vi "Simulation Statechart -DLL Wrapper.vi"(5 "firstStep?":bool, 7 "enableVisualization?":bool=TRUE, 8 "error in":errorcluster, 10 "sensors":T1 {"Kobuki Sensors"."Charger Source" items=["DISCHARGING"=0, "DOCKING_CHARGED"=2, "DOCKING_CHARGING"=6, "ADAPTER_CHARGED"=18, "ADAPTER_CHARGING"=22]; "accelerometer"."z axis (g)" format="%.3f"; "accelerometer"."y axis (g)" format="%.3f"; "accelerometer"."x axis (g)" format="%.3f"}) -> (0 "error out":errorcluster, 1 "Diagram Display":picture, 2 "sensors":T1 {"Kobuki Sensors"."Charger Source" items=["DISCHARGING"=0, "DOCKING_CHARGED"=2, "DOCKING_CHARGING"=6, "ADAPTER_CHARGED"=18, "ADAPTER_CHARGING"=22]; "accelerometer"."z axis (g)" format="%.3f"; "accelerometer"."y axis (g)" format="%.3f"; "accelerometer"."x axis (g)" format="%.3f"})   [LabVIEW 2015]
uses:
  shared/Accelerometer.ctl
  shared/Sensors.ctl
  Kobuki/Kobuki Bumps and WheelDrops.ctl
  Kobuki/Kobuki Buttons.ctl
  Kobuki/KobukiSensors.ctl
panel:
  # "Electrical: charging, battery, OI mode"
  # "Sensors: bump, cliff, button, wheel drop"
  # "Motors:"
  # "Inertia"
  # "Electrical: charging, battery, OI mode"
  # "Sensors: bump, cliff, button, wheel drop"
  # "Motors:"
  # "Inertia"
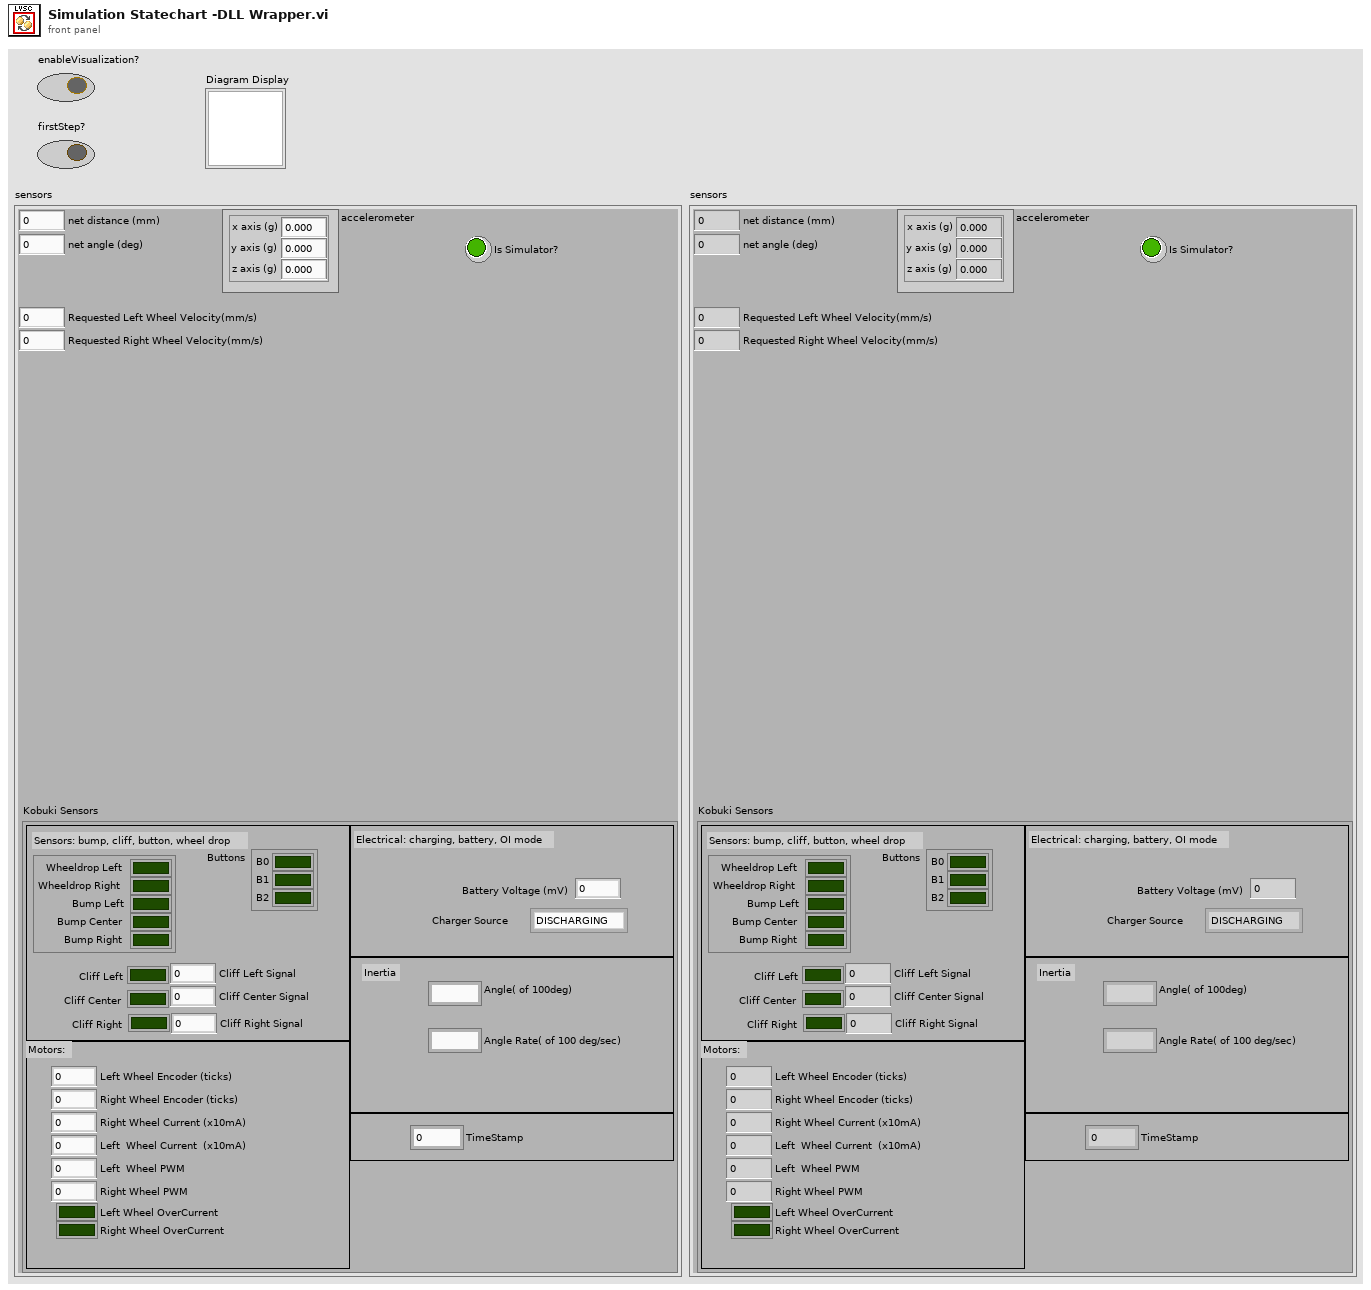
[diagram p1: front panel]
types:
  T1 = typedef "Sensors.ctl" = cluster{"net distance (mm)":i32, "net angle (deg)":i32, "accelerometer":T2, "Is Simulator?":bool, "Kobuki Sensors":T3, "Requested Left Wheel Velocity(mm/s)":i32, "Requested Right Wheel Velocity(mm/s)":i32}
  T2 = typedef "Accelerometer.ctl" = cluster{"x axis (g)":dbl, "y axis (g)":dbl, "z axis (g)":dbl}
  T3 = typedef "KobukiSensors.ctl" = cluster{"Bumps + Wheel Drops":T4, "Cliff Left":bool, "Cliff Center":bool, "Cliff Right":bool, "Cliff Left Signal":u16, "Cliff Center Signal":u16, "Cliff Right Signal":u16, "Buttons":T5, "Left Wheel Encoder (ticks)":u16, "Right Wheel Encoder (ticks) ":u16, "Left  Wheel PWM":i8, "Right Wheel PWM":i8, "Left Wheel OverCurrent":bool, "Right Wheel OverCurrent ":bool, "Right Wheel Current (x10mA)":i16, "Left  Wheel Current  (x10mA)":i16, "TimeStamp":u16, "Battery Voltage (mV)":i16, "Angle( of 100deg)":i16, "Angle Rate( of 100 deg/sec)":i16, "Charger Source ":i8}
  T4 = typedef "Kobuki Bumps and WheelDrops.ctl" = cluster{"Wheeldrop Left":bool, "Wheeldrop Right":bool, "Bump Left":bool, "Bump Center":bool, "Bump Right":bool}
  T5 = typedef "Kobuki Buttons.ctl" = cluster{"B0":bool, "B1":bool, "B2":bool}
  T6 = typedef "Sensor Group 6.ctl" = cluster{"Bumps + Wheel Drops":T7, "Wall":bool, "Cliff Left":bool, "Cliff Front Left":bool, "Cliff Front Right":bool, "Cliff Right":bool, "Wall Signal":u16, "Cliff Left Signal":u16, "Cliff Front Left Signal":u16, "Cliff Front Right Signal":u16, "Cliff Right Signal":u16, "Buttons":T8, "Virtual Wall":bool, "# Stream Packets":u8, "Requested Velocity (mm/s)":i16, "Requested Radius (mm)":i16, "Requested Right Wheel Velocity (mm/s)":i16, "Requested Left Wheel Velocity (mm/s)":i16, "Distance (mm)":i32, "Angle (deg)":i32, "Song Playing":bool, "Song Number":u8, "Charging State":T9, "Voltage (mV)":u16, "Current (mA)":i16, "Battery Temperature (deg C)":i8, "Battery Charge (mAh)":u16, "Battery Capacity (mAh)":u16, "Charging Sources":T10, "OI Mode":T11, "Digital Inputs":T12, "Drivers & Wheel Overcurrent":T13, "Analog Signal":u16, "Infrared":u8}
  T7 = typedef "Bumps + Wheel Drops.ctl" = cluster{"Wheeldrop Caster":bool, "Wheeldrop Left":bool, "Wheeldrop Right":bool, "Bump Left":bool, "Bump Right":bool}
  T8 = typedef "Buttons.ctl" = cluster{"Advance":bool, "Play":bool}
  T9 = typedef "Charging State.ctl" = enum16{"Not Charging", "Reconditioning Charging", "Full Charging", "Trickle Charging", "Waiting", "Charging Fault Condition"}
  T10 = typedef "Charging Sources Available.ctl" = cluster{"Internal Charger":bool, "Home Base":bool}
  T11 = typedef "OI Mode.ctl" = enum16{"Off", "Passive", "Safe", "Full"}
  T12 = typedef "Cargo Bay Digital Inputs.ctl" = cluster{"Digital Input 0":bool, "Digital Input 1":bool, "Digital Input 2":bool, "Digital Input 3":bool, "Device Detect":bool}
  T13 = typedef "Low-Side Driver + Wheel Overcurrent.ctl" = cluster{"Low-Side Driver 0":bool, "Low-Side Driver 1":bool, "Low-Side Driver 2":bool, "Left Wheel":bool, "Right Wheel":bool}
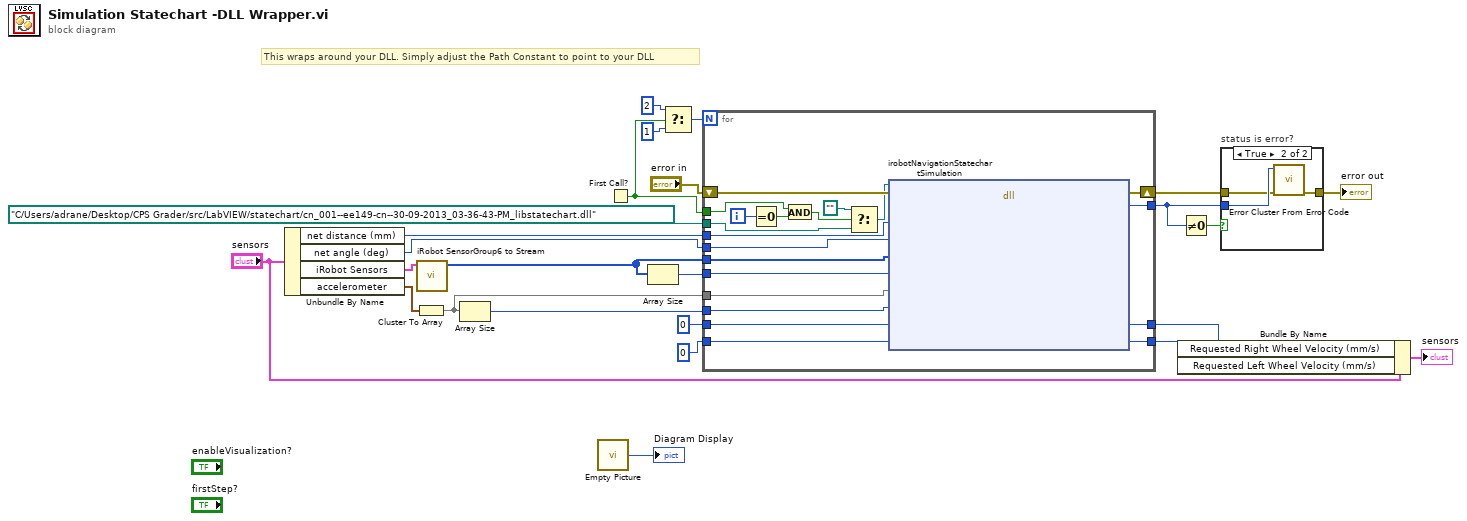
[diagram p0: block diagram]
diagram:
  # "This wraps around your DLL. Simply adjust the Path Constant to point to your DLL"
  n1 = Unbundle By Name("sensors") -> ("net distance (mm)"=w15:i32, "net angle (deg)"=w16:i32, "iRobot Sensors"=w23:T6, "accelerometer"=w24:T2)
  n2 = Cluster To Array(cluster=w24) -> (array=w19:dbl[])
  n3 = call "iRobot SensorGroup6 to Stream.vi"("iRobot Sensor Group 6"=w23) -> ("stream"=w17:u8[])  [unwired: 9 in, 1 out]
  n4 = Array Size(array=w19) -> (size(s)=w20:i32)
  n5 = call "Empty Picture"() -> ("empty picture"=→"Diagram Display":picture)
  n6 = First Call?() -> (First Call?: T/F=w2:bool)
  n7 = Array Size(array=w17) -> (size(s)=w18:i32)
  n8 = Select(t=2, s=w2, f=1) -> (s? t:f=w3:i32)
  n9 = for {
    N: w3 -> [_]
    tunnel: i16 0 ("rightWheelSpeed") -> [w45]
    tunnel: i16 0 ("rightWheelSpeed") -> [w44]
    tunnel: w20 -> [w43]
    tunnel: w19 -> [w42]
    tunnel: w18 -> [w41]
    tunnel: w17 -> [w40]
    tunnel: w16 -> [w39]
    tunnel: w15 -> [w38]
    tunnel: path "C:/Users/adrane/Desktop/CPS Grader/src/LabVIEW/statechart/cn_001--ee149-cn--30-09-2013_03-36-43-PM_libstatechart.dll" ("path in") -> [w32]
    tunnel: [w37] -> w12
    tunnel: [w36] -> w11
    tunnel: [w34] -> w8
    shift-right: [w35] -> w9
    shift-left: "error in" -> [w33]
    tunnel: w2 -> [w27]
    i -> [w29]
    n10 = Equal To 0?(x=w29) -> (x = 0?=w28:bool)
    n11 = And(x=w27, y=w28) -> (x .and. y?=w26:bool)
    n12 = Select(t=path "", s=w26, f=w32) -> (s? t:f=w31:path)
    n13 = dll-call lib="D:/Users/jjensen/workspace/Simulated iRobot Navigation/Release/libSimulated iRobot Navigation.dll" fn="irobotNavigationStatechartSimulation"(path in=w31, error in=w33, "netDistance"=w38, "netAngle"=w39, "sensorStream"=w40, "sensorStreamSize"=w41, "accelAxes"=w42, "accelAxesSize"=w43, "rightWheelSpeed"=w44, "leftWheelSpeed"=w45) -> (error out=w35:errorcluster, "status"=w34:i32, "rightWheelSpeed"=w37:i16, "leftWheelSpeed"=w36:i16)  [unwired: 7 in, 1 out]
  }
  n14 = Bundle By Name(cluster="sensors", "Requested Right Wheel Velocity (mm/s)"=w12, "Requested Left Wheel Velocity (mm/s)"=w11) -> (→"sensors":T1)
  n15 = Not Equal To 0?(x=w8) -> (x != 0?=w10:bool)
  n16 = case "status is error?" shown="True" w10 {
    tunnel: w8 -> [_ w49]
    tunnel: w9 -> [w46 w48]
    tunnel: [w46 w47] -> w6
    frame False {
    }
    frame True {
      n17 = call <vilib>:"Error Cluster From Error Code.vi"("error in (no error)"=w48, "error code (0)"=w49) -> ("error out"=w47:errorcluster)  [unwired: 7 in]
    }
  }
  "error out" <- w6
